vi "ConditionalUnsigned64.vi"(1 "Value in":u64) -> (0 "Stop?":bool)   [LabVIEW 2020]
doc: "Displays the value of the 64-bit unsigned integer numeric control and allows conditional breakpoints."
panel:
  in  "Tab Control":enum32{"Data   ", "Condition      "}(tab)
  out "Value":u64
  in  "Ls":u64
  in  "Gr":u64
  in  "Eq":u64
  in  "Ls":bool
  in  "Gr":bool
  in  "Eq":bool
  # "Pause if any of the following:"
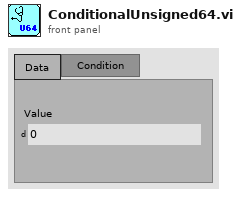
[diagram p1: front panel]
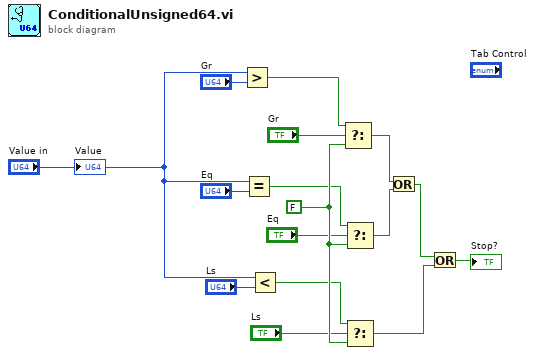
[diagram p0: block diagram]
diagram:
  w13 = FALSE ("f")
  n1 = Greater?(x="Value in", y="Gr") -> (0:w1:bool)
  n2 = Equal?(x="Value in", y="Eq") -> (x = y?=w10:bool)
  n3 = Less?(x="Value in", y="Ls") -> (x < y?=w3:bool)
  n4 = Select(t=w1, s="Gr", f=w13) -> (s? t:f=w7:bool)
  n5 = Select(t=w10, s="Eq", f=w13) -> (s? t:f=w6:bool)
  n6 = Select(t=w3, s="Ls", f=w13) -> (s? t:f=w4:bool)
  n7 = Or(x=w7, y=w6) -> (x .or. y?=w5:bool)
  n8 = Or(x=w5, y=w4) -> (x .or. y?=→"Stop?":bool)
  "Value" <- "Value in"
